vi "Get Control References.vi"(3 "error in":errorcluster, 5 "VI  Ref":refnum<vi>) -> (0 "error out":errorcluster, 1 "Control Names":string[](array[string]), 2 "Controls[]":refnum<vi>[](array[refnum]))   [LabVIEW 2019]
doc: "Returns an array of control references and a string array of control label names, from the front panel of the calling VI.\n\nThis VI also accounts for tab controls within other tab controls."
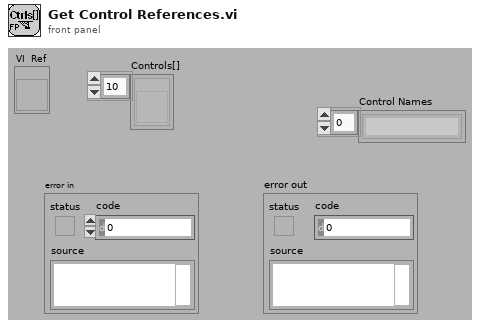
[diagram p1: front panel]
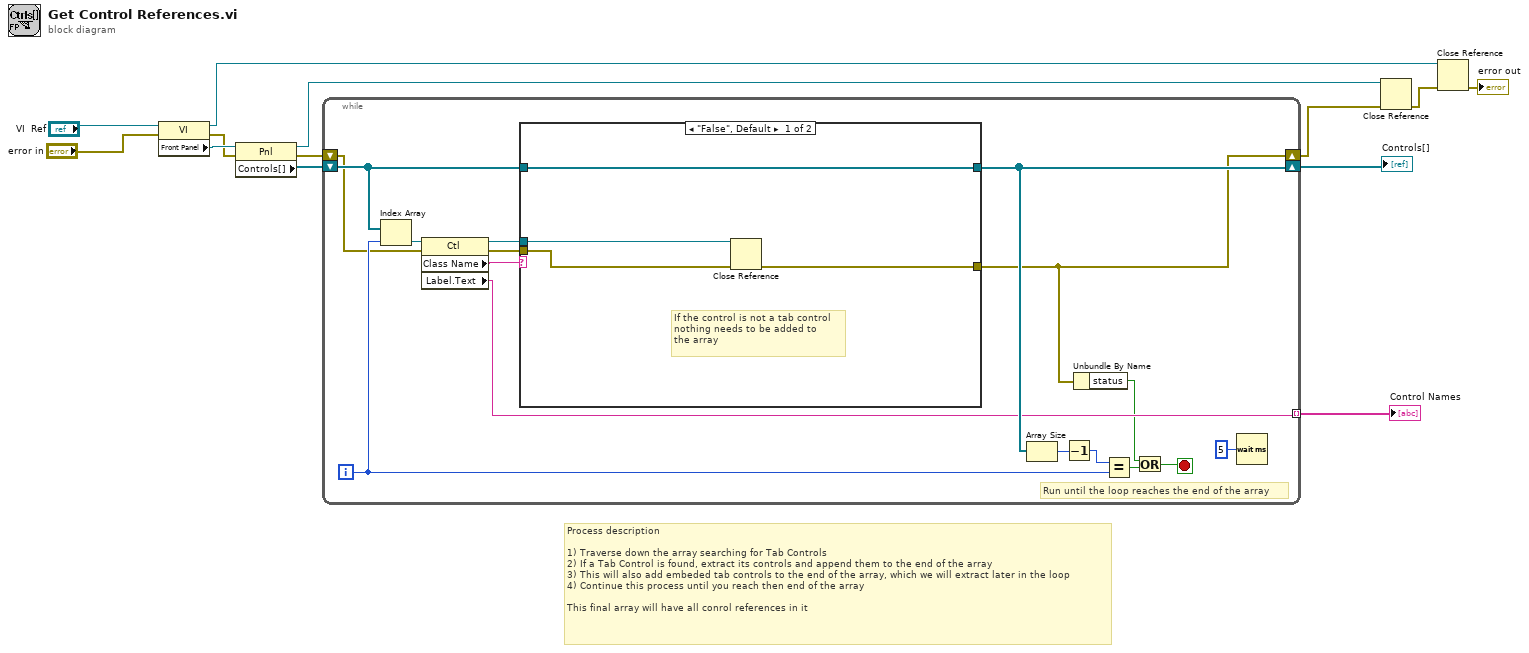
[diagram p0: block diagram]
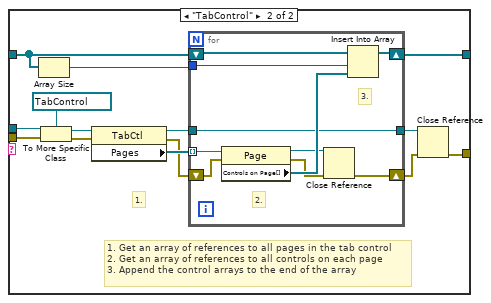
[diagram p2: hidden frame]
diagram:
  # "Process description\n\n1) Traverse down the array searching for Tab Controls\n2) If a Tab Control is found, extract its controls and append them to the end of the array\n3) This will also add embeded tab controls to the end of the array, which we will extract later in the loop\n4) Continue this process until you reach then end of the array\n\nThis final array will have all conrol references in it"
  n1 = property class="VI"(reference="VI  Ref", error in="error in") -> (reference out=w7:refnum<vi>, error out=w9:errorcluster, "Front Panel"=w10:refnum<vi>)
  n2 = property class="Pnl"(reference=w10, error in=w9) -> (reference out=w6:refnum<vi>, error out=w8:errorcluster, "Controls[]"=w11:refnum<vi>[])
  n3 = while {
    shift-right: [w21] -> w12
    shift-left: w11 -> [w27]
    tunnel: [w18] -> w13 mode=indexing
    shift-right: [w17] -> w4
    shift-left: w8 -> [w20]
    i -> [w22]
    stop <- w15 stop-if-true
    # "Run until the loop reaches the end of the array"
    n4 = Index Array(array=w27, index=w22) -> (element=w23:refnum<vi>)
    n5 = property class="Ctl"(reference=w23, error in=w20) -> (reference out=w28:refnum<vi>, error out=w19:errorcluster, "Class Name"=w26:string, "Label.Text"=w18:string)
    n6 = case shown="\"False\", Default" w26 {
      tunnel: w28 -> [w32 w47]
      tunnel: w27 -> [w33 w43]
      tunnel: [w33 w44] -> w21
      tunnel: w19 -> [w31 w40]
      tunnel: [w30 w36] -> w17
      frame "False", Default {
        # "If the control is not a tab control\nnothing needs to be added to\nthe array"
        n7 = Close Reference(reference=w32, error in (no error)=w31) -> (error out=w30:errorcluster)
      }
      frame "TabControl" {
        # "1. Get an array of references to all pages in the tab control\n2. Get an array of references to all controls on each page\n3. Append the control arrays to the end of the array"
        # "1."
        n8 = Array Size(array=w43) -> (size(s)=w41:i32)
        n9 = To More Specific Class(target class=refnum<vi> refnum ("Tab Control"), reference=w47, error in=w40) -> (specific class reference=w46:refnum<vi>, error out=w39:errorcluster)
        n10 = property class="TabCtl"(reference=w46, error in=w39) -> (reference out=w37:refnum<vi>, error out=w38:errorcluster, "Pages"=w45:refnum<vi>[])
        n11 = for {
          tunnel: w45 -> [w57] mode=indexing
          tunnel: w41 -> [w55]
          shift-right: [w56] -> w44
          shift-left: w43 -> [w54]
          tunnel: w37 -> [w51]
          tunnel: [w51] -> w35
          shift-right: [w48] -> w34
          shift-left: w38 -> [w52]
          # "3."
          # "2."
          n12 = property class="Page"(reference=w57, error in=w52) -> (reference out=w50:refnum<vi>, error out=w49:errorcluster, "Controls on Page[]"=w53:refnum<vi>[])
          n13 = Close Reference(reference=w50, error in (no error)=w49) -> (error out=w48:errorcluster)
          n14 = Insert Into Array(array=w54, index=w55, new element=w53) -> (w56:refnum<vi>[])
        }
        n15 = Close Reference(reference=w35, error in (no error)=w34) -> (error out=w36:errorcluster)
      }
    }
    n16 = Array Size(array=w21) -> (size(s)=w25:i32)
    n17 = Decrement(x=w25) -> (x-1=w24:i32)
    n18 = Unbundle By Name(w17) -> ("status"=w14:bool)
    n19 = Equal?(x=w24, y=w22) -> (x = y?=w16:bool)
    n20 = Or(x=w14, y=w16) -> (x .or. y?=w15:bool)
    n21 = Wait (ms)(milliseconds to wait=u32 5) -> ()  [unwired: 1 out]
  }
  "Control Names" <- w13
  "Controls[]" <- w12
  n22 = Close Reference(reference=w6, error in (no error)=w4) -> (error out=w5:errorcluster)
  n23 = Close Reference(reference=w7, error in (no error)=w5) -> (error out=→"error out":errorcluster)
